vi "Add Configurations Section.vi"(7 "Control references":refnum<vi>[](array[refnum]), 8 "error in":errorcluster, 11 "File refnum in":refnum<file>) -> (0 "error out":errorcluster, 3 "File refnum out":refnum<file>)   [LabVIEW 2021]
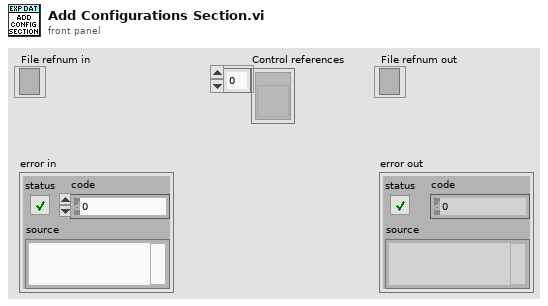
[diagram p1: front panel]
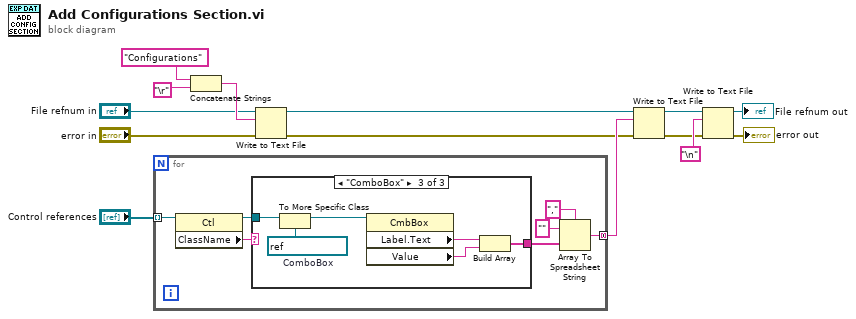
[diagram p0: block diagram]
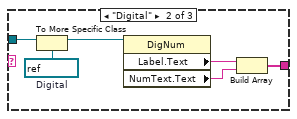
[diagram p3: hidden frame]
diagram:
  n1 = for {
    tunnel: "Control references" -> [w20] mode=indexing
    tunnel: [w15] -> w7 mode=concatenating
    n2 = property class="Ctl"(reference=w20) -> (reference out=w21:refnum<vi>, "ClassName"=w19:string)  [unwired: 1 in, 1 out]
    n3 = case shown="\"ComboBox\"" w19 {
      tunnel: w21 -> [_ w24 w30]
      tunnel: [_ w22 w28] -> w17
      frame Default {
      }
      frame "Digital" {
        w23 = refnum<vi> refnum  # Digital
        n4 = To More Specific Class(target class=w23, reference=w24) -> (specific class reference=w25:refnum<vi>)  [unwired: 1 in, 1 out]
        n5 = property class="DigNum"(reference=w25) -> ("Label.Text"=w27:string, "NumText.Text"=w26:string)  [unwired: 1 in, 2 out]
        n6 = Build Array(w27, w26) -> (w22:string[])
      }
      frame "ComboBox" {
        w29 = refnum<vi> refnum  # ComboBox
        n7 = To More Specific Class(target class=w29, reference=w30) -> (specific class reference=w31:refnum<vi>)  [unwired: 1 in, 1 out]
        n8 = property class="CmbBox"(reference=w31) -> ("Label.Text"=w33:string, "Value"=w32:string)  [unwired: 1 in, 2 out]
        n9 = Build Array(w33, w32) -> (w28:string[])
      }
    }
    n10 = Array To Spreadsheet String(delimiter (Tab)=",", array=w17, 3:"" ("format string")) -> (spreadsheet string=w15:string)
  }
  n11 = Concatenate Strings("Configurations" ("format string"), "\r") -> (w12:string)
  n12 = Write to Text File(file (use dialog)="File refnum in", text=w12, error in="error in") -> (refnum out=w6:refnum<file>, error out=w4:errorcluster)  [unwired: 1 in, 1 out]
  n13 = Write to Text File(file (use dialog)=w6, text=w7, error in=w4) -> (refnum out=w5:refnum<file>, error out=w3:errorcluster)  [unwired: 1 in, 1 out]
  n14 = Write to Text File(file (use dialog)=w5, text="\n", error in=w3) -> (refnum out=→"File refnum out":refnum<file>, error out=→"error out":errorcluster)  [unwired: 1 in, 1 out]
